vi "ELConverter.vi"(1 "ELdata: All Data":string="1081000005ff0102900161018000") -> (0 "JSON":string)   [LabVIEW 2017]
uses:
  <vilib>/httpClient/LabVIEWHTTPClient.lvlib
panel:
  out "error out":errorcluster
  out "requestUriString":string
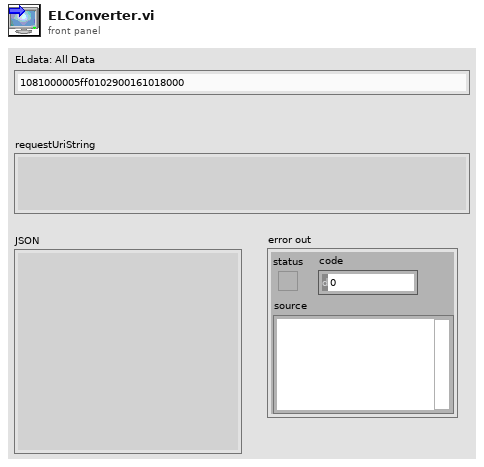
[diagram p1: front panel]
types:
  T1 = typedef "LabVIEWHTTPClient.lvlib/ClientHandle.ctl" = refnum<k1>
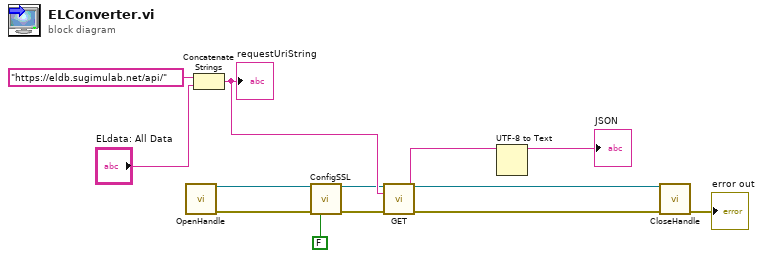
[diagram p0: block diagram]
diagram:
  n1 = call <vilib>:"OpenHandle.vi"() -> ("client handle out"=w4:T1, "error out"=w5:errorcluster)  [unwired: 14 in]
  n2 = Concatenate Strings("https://eldb.sugimulab.net/api/", "ELdata: All Data") -> (w8:string)
  "requestUriString" <- w8
  n3 = call <vilib>:"ConfigSSL.vi"("client handle"=w4, "error in (no error)"=w5, "verify server (true)"=FALSE) -> ("client handle out"=w7:T1, "error out"=w6:errorcluster)  [unwired: 11 in]
  n4 = call <vilib>:"GET.vi"("client handle"=w7, "url"=w8, "error in (no error)"=w6) -> ("client handle out"=w11:T1, "body"=w1:string, "error out"=w10:errorcluster)  [unwired: 9 in, 1 out]
  n5 = UTF-8 to Text(11:w1) -> (3:→"JSON":string)  [unwired: 2 in, 1 out]
  n6 = call <vilib>:"CloseHandle.vi"("client handle"=w11, "error in (no error)"=w10) -> ("error out"=→"error out":errorcluster)  [unwired: 13 in]
